vi "pockelscontrol_goMD.vi"() -> ()   [LabVIEW 2012]
doc: "SciScan 1.2 160622"
uses:
  GFG/GFGfpRefGet.vi
  GFG/GFGnumericGet.vi
  GFG/GFGbooleanGet.vi
  GFG/GFGstringGet.vi
  <vilib>/DAQmx/create/channels.llb/DAQmx Create Channel (AO-Voltage-Basic).vi
  <vilib>/DAQmx/write.llb/DAQmx Write (Analog DBL 1Chan 1Samp).vi
  GFG/GFG library.lvlib
panel:
  out "error out 3":errorcluster
  out "error out 2":errorcluster
  out "error out":errorcluster
  out "Source VI":string
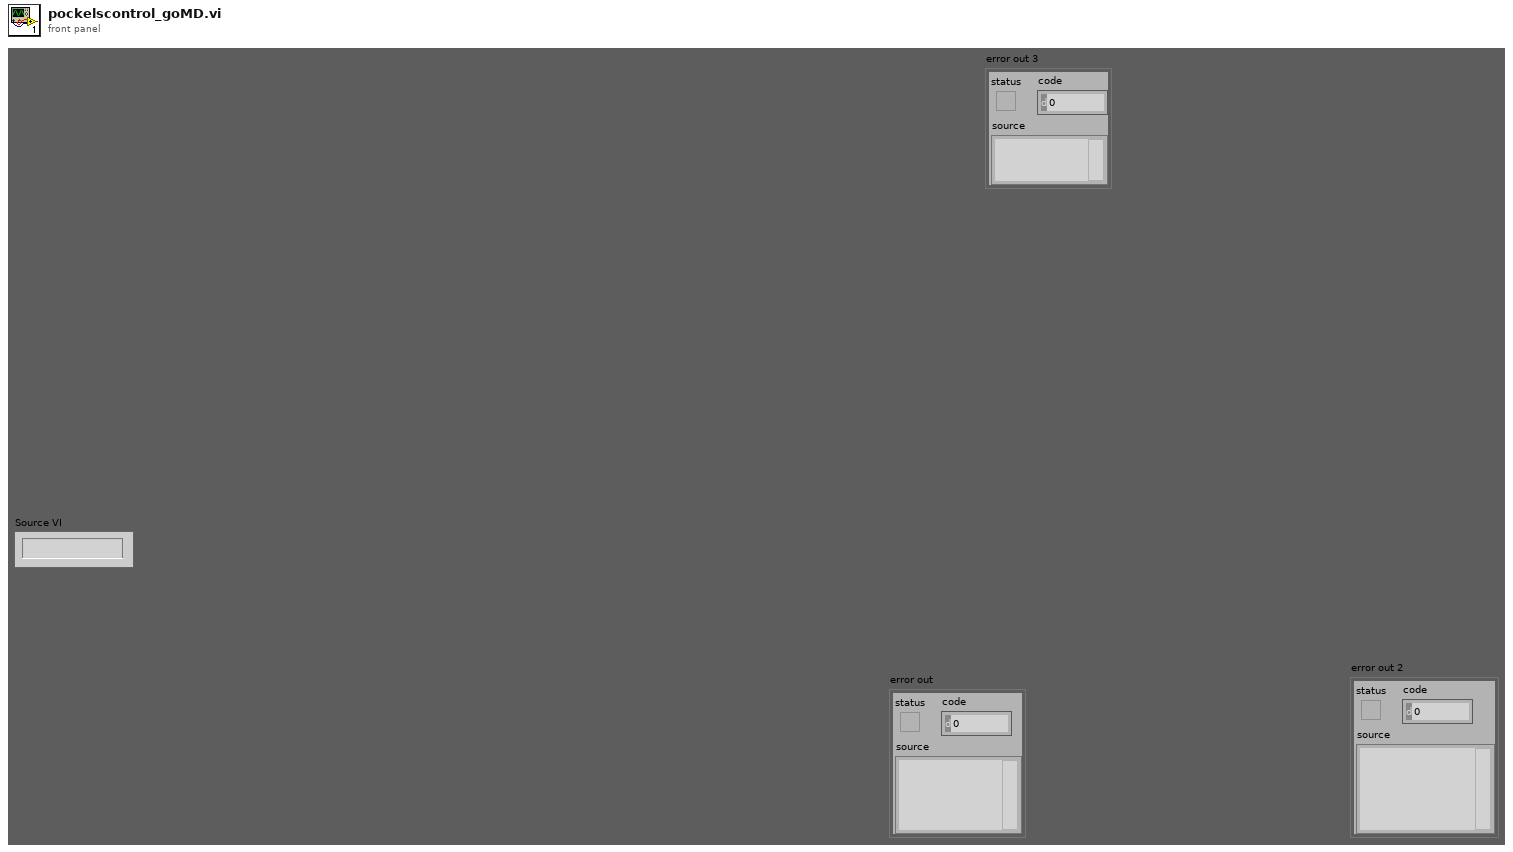
[diagram p1: front panel]
types:
  T1 = enum8{"Enabled", "Disabled", "Disabled and Grayed Out"}
  T2 = cluster{"WaveformChartRef":refnum<vi>, "DigitalRef":refnum<vi>, "ArrayRef":refnum<vi>, "TabControlRef":refnum<vi>, "EnumRef":refnum<vi>, "RingRef":refnum<vi>, "BooleanRef":refnum<vi>, "KnobRef":refnum<vi>, "SlideRef":refnum<vi>, "PathRef":refnum<vi>, "StringRef":refnum<vi>, "ComboBox":refnum<vi>, "WaveformGraphRef":refnum<vi>}
  T3 = enum16{"Left Button", "Center Button", "Right Button", "Window Close"}
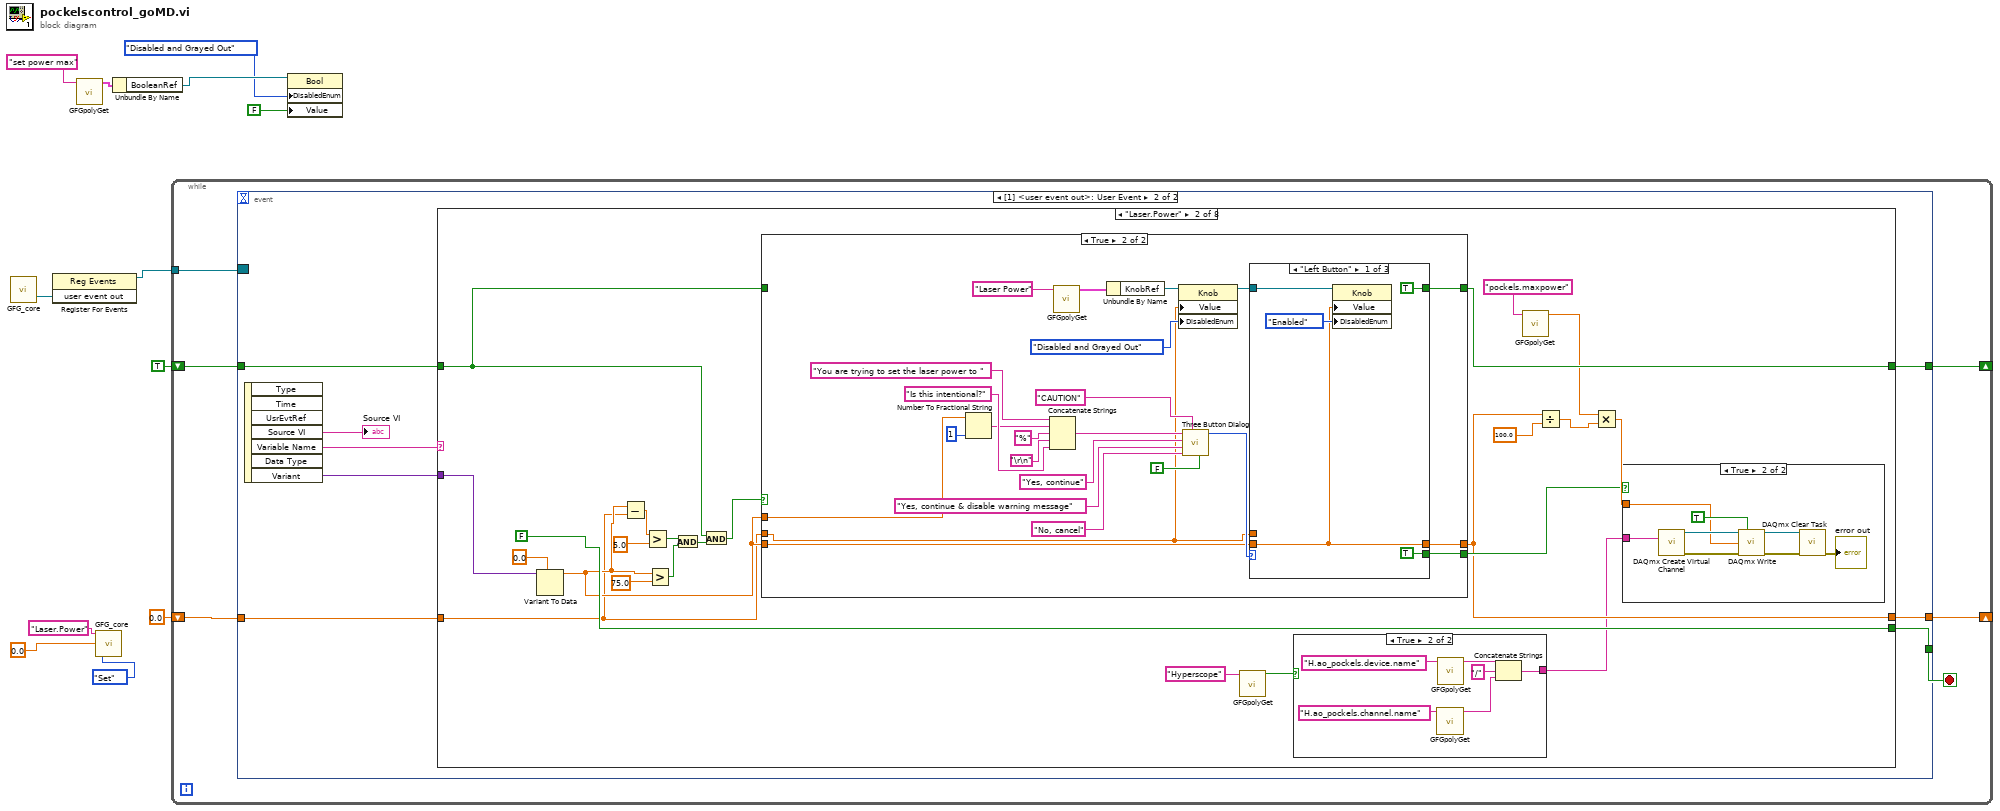
[diagram p0: block diagram]
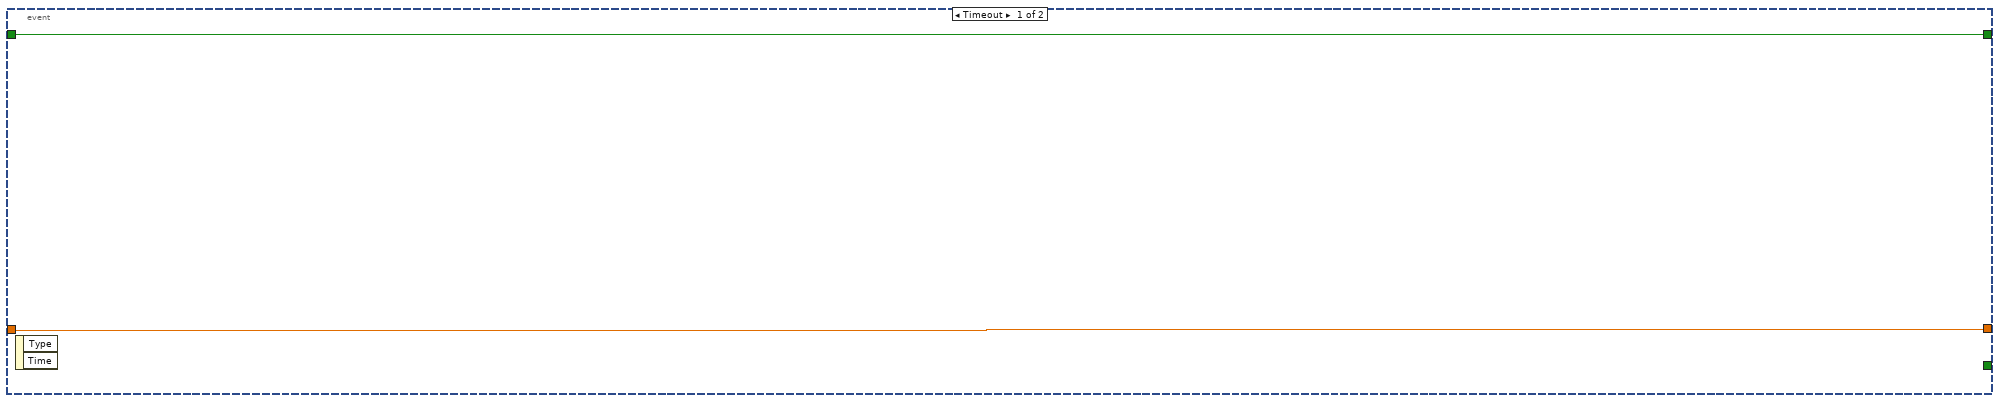
[diagram p2: hidden frame]
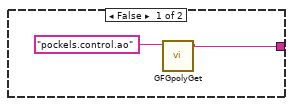
[diagram p4: hidden frame]
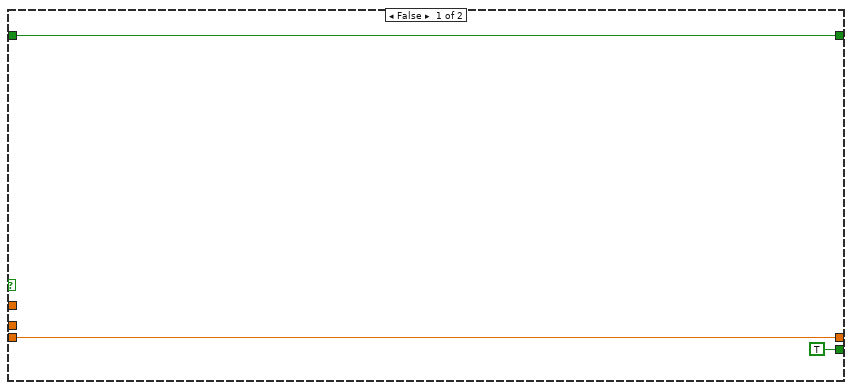
[diagram p5: hidden frame]
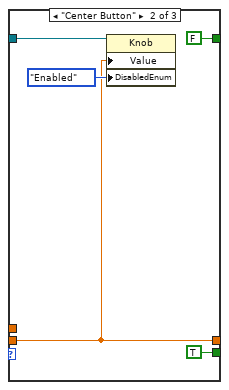
[diagram p6: hidden frame]
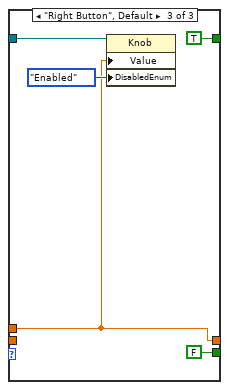
[diagram p7: hidden frame]
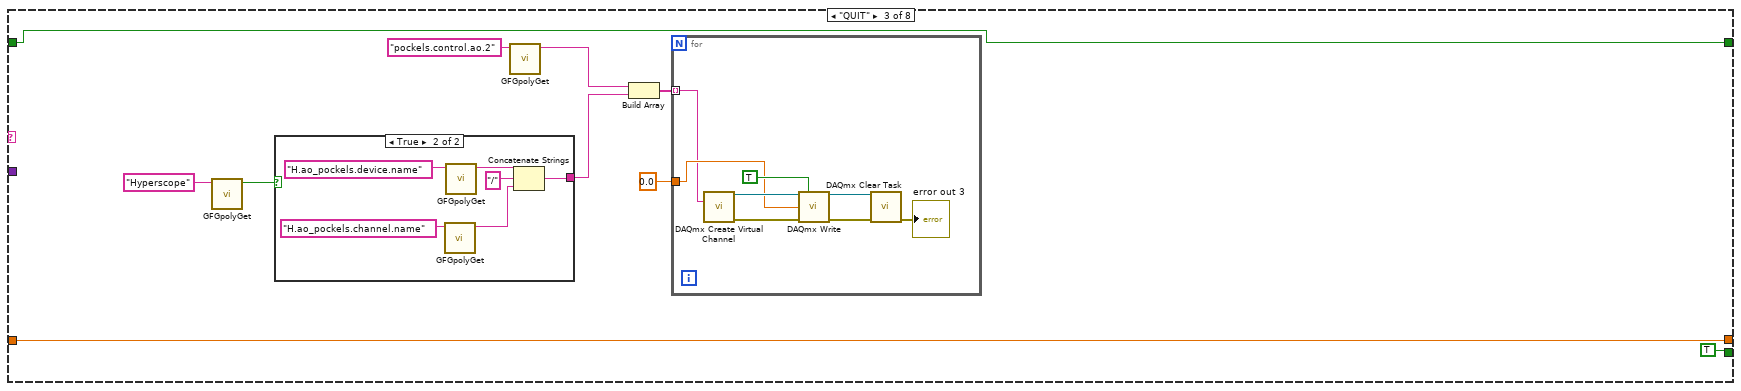
[diagram p9: hidden frame]
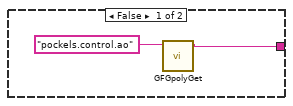
[diagram p10: hidden frame]
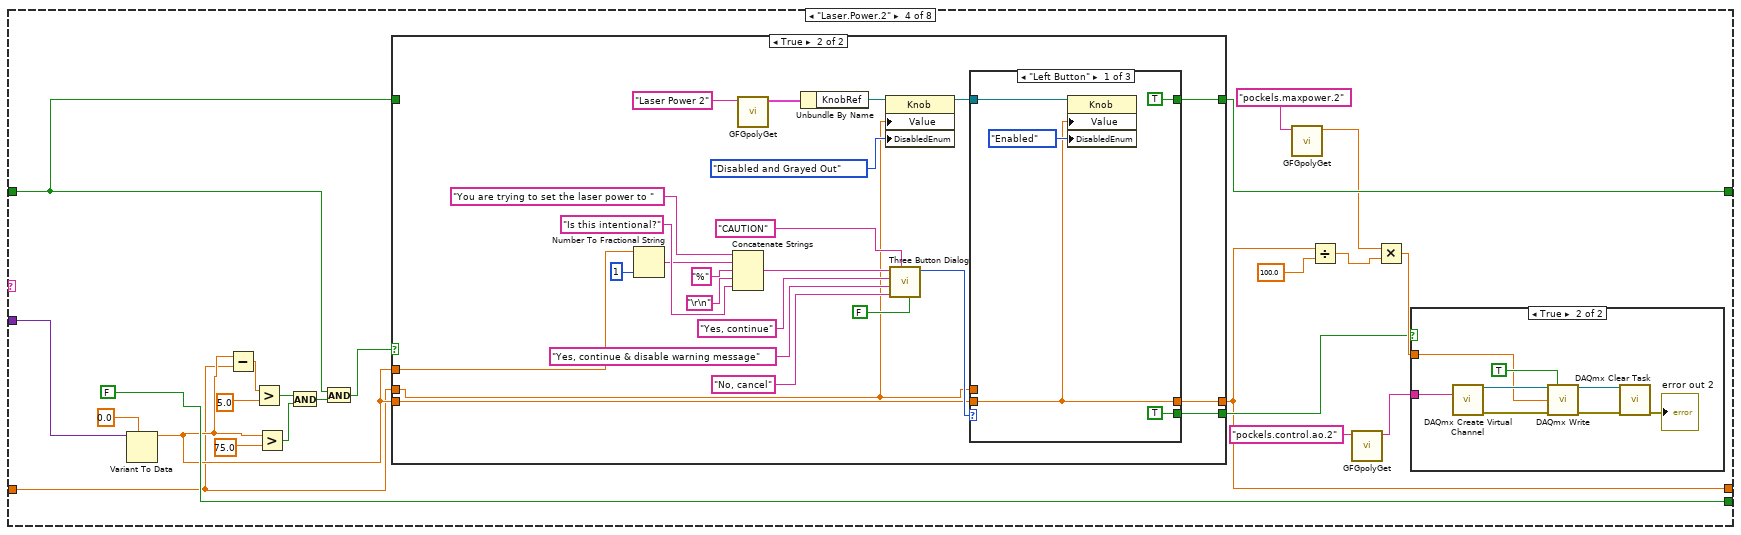
[diagram p11: hidden frame]
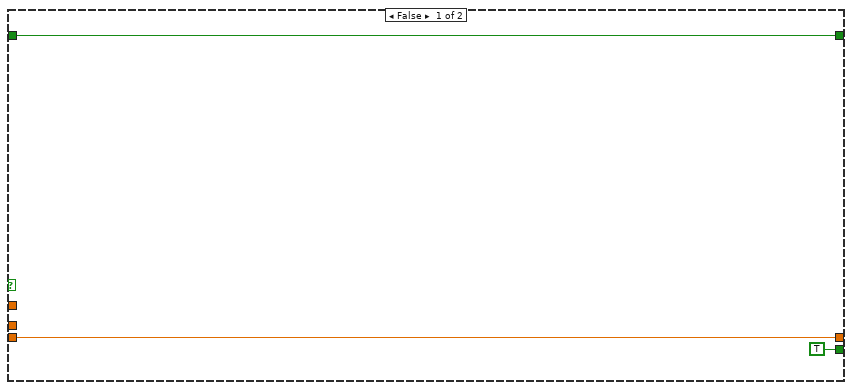
[diagram p12: hidden frame]
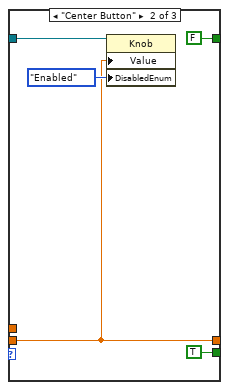
[diagram p13: hidden frame]
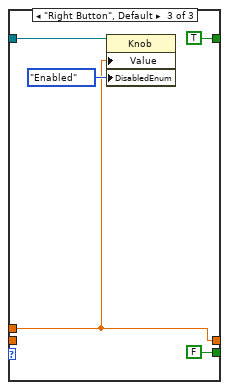
[diagram p14: hidden frame]
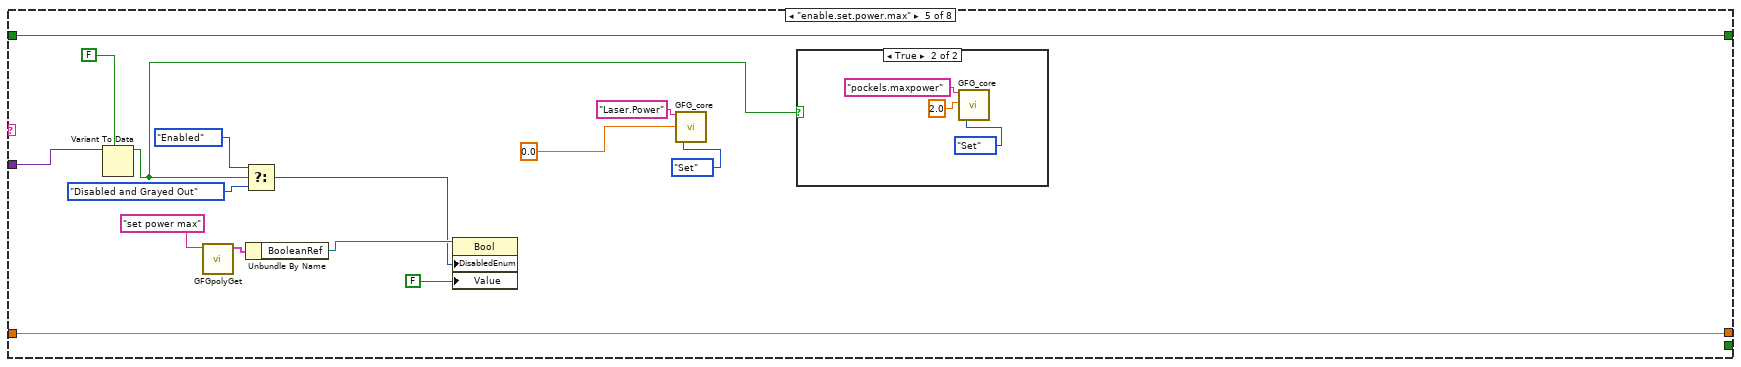
[diagram p16: hidden frame]
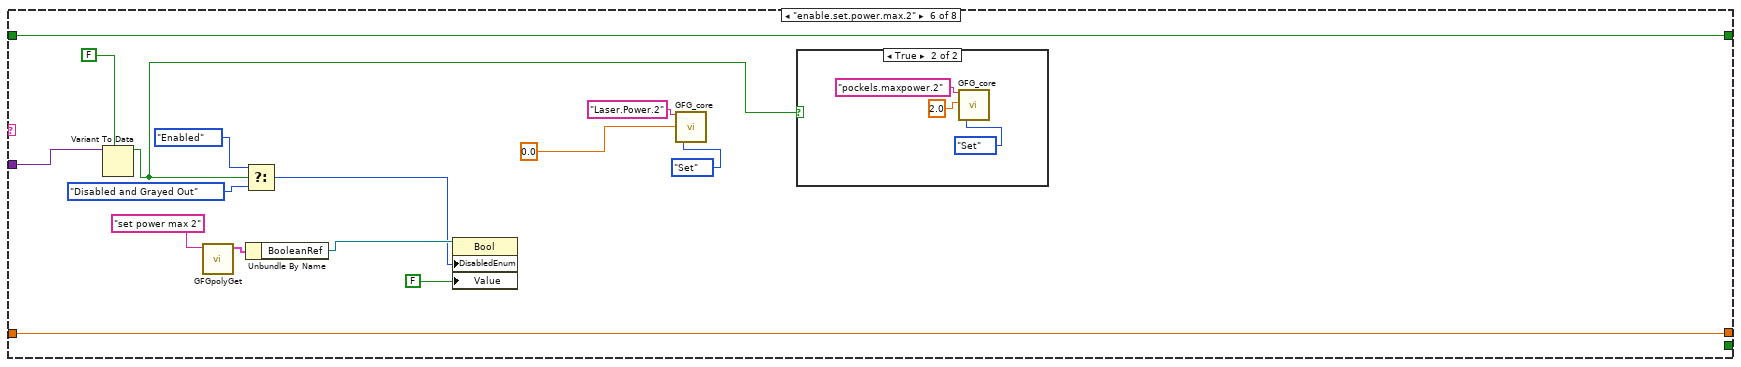
[diagram p18: hidden frame]
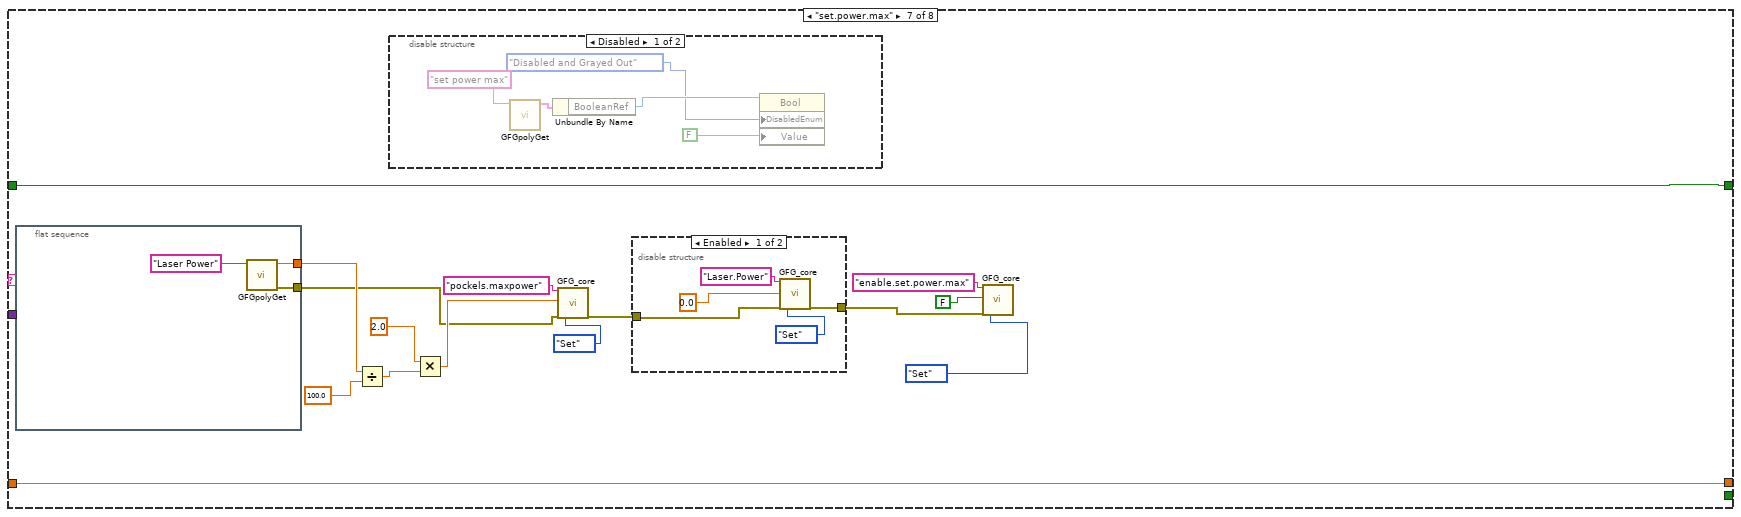
[diagram p20: hidden frame]
diagram:
  n1 = call "GFG_core.vi"() -> ("user event out"=w12:refnum<user-event>)  [unwired: 13 in, 6 out]
  n2 = register-events(w12) -> (reference out=w11:refnum<event-registration>)  [unwired: 2 in, 1 out]
  n3 = call-poly "GFGpolyGet.vi"("Variable Name in"="set power max") -> ("output cluster"=w3:T2)  [unwired: 9 in, 1 out]
  n4 = call "GFG_core.vi"("Variable Name in"="Laser.Power", "Variant in"=0.0 ("Laser Power"), "Action"=enum16{"Init", "Set", "Get"}."Set") -> ()  [unwired: 10 in, 7 out]
  n5 = Unbundle By Name(w3) -> ("BooleanRef"=w4:refnum<vi>)
  n6 = while {
    tunnel: w11 -> [w18]
    shift-right: [w16] -> _
    shift-left: 0.0 ("Laser Power") -> [w15]
    shift-right: [w14] -> _
    shift-left: TRUE -> [w13]
    stop <- w17 stop-if-true
    n7 = event shown="[1] <user event out>: User Event" {
      selector: w18 -> [_ _]
      dyn-events: _ -> [_ _]
      timeout: _ -> [_ _]
      tunnel: [_ w25] -> w17
      tunnel: [w20 w24] -> w16
      tunnel: w15 -> [w20 w23]
      tunnel: [w19 w22] -> w14
      tunnel: w13 -> [w19 w21]
      event Timeout {
        n8 = event-data() -> ()  [unwired: 1 in, 2 out]
      }
      event User Event {
        n9 = event-data() -> ("Source VI"=→"Source VI":string, "Variable Name"=w28:string, "Variant"=w27:variant)  [unwired: 1 in, 4 out]
        n10 = case shown="\"Laser.Power\"" w28 {
          tunnel: w27 -> [_ w54 _ w161 w218 w236 _ _]
          tunnel: [_ FALSE TRUE FALSE _ _ _ _] -> w25
          tunnel: [w30 w43 w117 w150 w223 w241 w262 w290] -> w24
          tunnel: w23 -> [w30 w40 w117 w147 w223 w241 w262 w290]
          tunnel: [w29 w46 w116 w153 w222 w240 w261 w289] -> w22
          tunnel: w21 -> [w29 w44 w116 w151 w222 w240 w261 w289]
          frame "False", Default {
          }
          frame "Laser.Power" {
            n11 = Variant To Data(type=0.0 ("Laser Power"), Variant=w54) -> (data=w41:dbl)  [unwired: 1 in, 1 out]
            n12 = Subtract(x=w41, y=w40) -> (x-y=w39:dbl)
            n13 = Greater?(x=w39, y=5.0) -> (0:w37:bool)
            n14 = Greater?(x=w41, y=75.0) -> (0:w49:bool)
            n15 = And(x=w37, y=w49) -> (x .and. y?=w42:bool)
            n16 = And(x=w44, y=w42) -> (x .and. y?=w45:bool)
            n17 = case shown="True" w45 {
              tunnel: [TRUE w83] -> w47
              tunnel: [w64 w82] -> w46
              tunnel: w44 -> [w64 _]
              tunnel: w40 -> [_ w70]
              tunnel: w41 -> [_ w80]
              tunnel: w41 -> [w63 w71]
              tunnel: [w63 w66] -> w43
              frame False {
              }
              frame True {
                n18 = Number To Fractional String(number=w80, precision (6)=i16 1) -> (F-format string=w69:string)  [unwired: 2 in]
                n19 = Concatenate Strings("You are trying to set the laser power to " ("message"), w69, "%" ("string"), "\r\n", "Is this intentional?" ("string")) -> (w77:string)
                n20 = call-poly "GFGpolyGet.vi"("Variable Name in"="Laser Power") -> ("output cluster"=w75:T2)  [unwired: 9 in, 1 out]
                n21 = Unbundle By Name(w75) -> ("KnobRef"=w74:refnum<vi>)
                n22 = property class="Knob"(reference=w74, "Value"=w70, "DisabledEnum"=T1."Disabled and Grayed Out" ("Disabled")) -> (reference out=w72:refnum<vi>)  [unwired: 1 in, 1 out]
                n23 = call <vilib>:"Three Button Dialog.vi"("Allow user to close window? (TRUE)"=FALSE, "Window Title (\"\")"="CAUTION" ("Window Title (\"\")"), "Right Button Text (\"Cancel\")"="No, cancel" ("Right Button Text (\"Cancel\")"), "Center Button Text (\"No\")"="Yes, continue & disable warning message" ("Center Button Text (\"No\")"), "Left Button Text (\"Yes\")"="Yes, continue" ("Left Button Text (\"Yes\")"), "message"=w77) -> ("Which Button?"=w84:T3)  [unwired: 5 in]
                n24 = case shown="\"Left Button\"" w84 {
                  tunnel: [TRUE TRUE FALSE] -> w83
                  tunnel: [TRUE FALSE TRUE] -> w82
                  tunnel: w72 -> [w91 w96 w101]
                  tunnel: w71 -> [w90 w95 _]
                  tunnel: w70 -> [_ _ w100]
                  tunnel: [w90 w95 w100] -> w66
                  frame "Left Button" {
                    n25 = property class="Knob"(reference=w91, "Value"=w90, "DisabledEnum"=T1."Enabled" ("Disabled")) -> ()  [unwired: 1 in, 2 out]
                  }
                  frame "Center Button" {
                    n26 = property class="Knob"(reference=w96, "Value"=w95, "DisabledEnum"=T1."Enabled" ("Disabled")) -> ()  [unwired: 1 in, 2 out]
                  }
                  frame "Right Button", Default {
                    n27 = property class="Knob"(reference=w101, "Value"=w100, "DisabledEnum"=T1."Enabled" ("Disabled")) -> ()  [unwired: 1 in, 2 out]
                  }
                }
              }
            }
            n28 = call-poly "GFGpolyGet.vi"("Variable Name in"="Hyperscope") -> ("Boolean Value OUT"=w31:bool)  [unwired: 9 in, 1 out]
            n29 = case shown="True" w31 {
              tunnel: [w55 w57] -> w32
              frame False {
                n30 = call-poly "GFGpolyGet.vi"("Variable Name in"="pockels.control.ao" ("Tag in")) -> ("String"=w55:string)  [unwired: 9 in, 1 out]
              }
              frame True {
                n31 = call-poly "GFGpolyGet.vi"("Variable Name in"="H.ao_pockels.channel.name" ("Tag in")) -> ("String"=w58:string)  [unwired: 9 in, 1 out]
                n32 = call-poly "GFGpolyGet.vi"("Variable Name in"="H.ao_pockels.device.name" ("Tag in")) -> ("String"=w61:string)  [unwired: 9 in, 1 out]
                n33 = Concatenate Strings(w61, "/" ("Variable Name in"), w58) -> (w57:string)
              }
            }
            n34 = call-poly "GFGpolyGet.vi"("Variable Name in"="pockels.maxpower") -> ("Numeric"=w35:dbl)  [unwired: 8 in, 2 out]
            n35 = Divide(x=w43, y=100.0 ("x")) -> (x/y=w52:dbl)
            n36 = Multiply(x=w35, y=w52) -> (x*y=w50:dbl)
            n37 = case shown="True" w47 {
              tunnel: w32 -> [_ w112]
              tunnel: w50 -> [_ w106]
              frame False {
              }
              frame True {
                n38 = call-poly <vilib>:"DAQmx Create Virtual Channel.vi"("physical channels"=w112) -> ("task out"=w111:refnum<k21>, "error out"=w107:errorcluster)  [unwired: 13 in]
                n39 = call-poly <vilib>:"DAQmx Write.vi"("task/channels in"=w111, "auto start"=TRUE, "data"=w106, "error in"=w107) -> ("task out"=w109:refnum<k21>, "error out"=w108:errorcluster)  [unwired: 9 in, 1 out]
                n40 = call <vilib>:"DAQmx Clear Task.vi"("task in"=w109, "error in"=w108) -> ("error out"=→"error out":errorcluster)  [unwired: 13 in]
              }
            }
          }
          frame "QUIT" {
            n41 = call-poly "GFGpolyGet.vi"("Variable Name in"="Hyperscope") -> ("Boolean Value OUT"=w113:bool)  [unwired: 9 in, 1 out]
            n42 = case shown="True" w113 {
              tunnel: [w123 w125] -> w114
              frame False {
                n43 = call-poly "GFGpolyGet.vi"("Variable Name in"="pockels.control.ao" ("Tag in")) -> ("String"=w123:string)  [unwired: 9 in, 1 out]
              }
              frame True {
                n44 = call-poly "GFGpolyGet.vi"("Variable Name in"="H.ao_pockels.channel.name" ("Tag in")) -> ("String"=w126:string)  [unwired: 9 in, 1 out]
                n45 = call-poly "GFGpolyGet.vi"("Variable Name in"="H.ao_pockels.device.name" ("Tag in")) -> ("String"=w129:string)  [unwired: 9 in, 1 out]
                n46 = Concatenate Strings(w129, "/" ("Variable Name in"), w126) -> (w125:string)
              }
            }
            n47 = call-poly "GFGpolyGet.vi"("Variable Name in"="pockels.control.ao.2" ("Tag in")) -> ("String"=w120:string)  [unwired: 9 in, 1 out]
            n48 = Build Array(w120, w114) -> (w119:string[])
            n49 = for {
              tunnel: 0.0 ("data") -> [w132]
              tunnel: w119 -> [w131] mode=indexing
              n50 = call-poly <vilib>:"DAQmx Create Virtual Channel.vi"("physical channels"=w131) -> ("task out"=w138:refnum<k21>, "error out"=w134:errorcluster)  [unwired: 13 in]
              n51 = call-poly <vilib>:"DAQmx Write.vi"("task/channels in"=w138, "auto start"=TRUE, "data"=w132, "error in"=w134) -> ("task out"=w136:refnum<k21>, "error out"=w135:errorcluster)  [unwired: 9 in, 1 out]
              n52 = call <vilib>:"DAQmx Clear Task.vi"("task in"=w136, "error in"=w135) -> ("error out"=→"error out 3":errorcluster)  [unwired: 13 in]
            }
          }
          frame "Laser.Power.2" {
            n53 = Variant To Data(type=0.0 ("Laser Power"), Variant=w161) -> (data=w148:dbl)  [unwired: 1 in, 1 out]
            n54 = Subtract(x=w148, y=w147) -> (x-y=w146:dbl)
            n55 = Greater?(x=w146, y=5.0) -> (0:w144:bool)
            n56 = Greater?(x=w148, y=75.0) -> (0:w156:bool)
            n57 = And(x=w144, y=w156) -> (x .and. y?=w149:bool)
            n58 = And(x=w151, y=w149) -> (x .and. y?=w152:bool)
            n59 = case shown="True" w152 {
              tunnel: [TRUE w182] -> w154
              tunnel: [w163 w181] -> w153
              tunnel: w151 -> [w163 _]
              tunnel: w147 -> [_ w169]
              tunnel: w148 -> [_ w179]
              tunnel: w148 -> [w162 w170]
              tunnel: [w162 w165] -> w150
              frame False {
              }
              frame True {
                n60 = Number To Fractional String(number=w179, precision (6)=i16 1) -> (F-format string=w168:string)  [unwired: 2 in]
                n61 = Concatenate Strings("You are trying to set the laser power to " ("message"), w168, "%" ("string"), "\r\n", "Is this intentional?" ("string")) -> (w176:string)
                n62 = call-poly "GFGpolyGet.vi"("Variable Name in"="Laser Power 2") -> ("output cluster"=w174:T2)  [unwired: 9 in, 1 out]
                n63 = Unbundle By Name(w174) -> ("KnobRef"=w173:refnum<vi>)
                n64 = property class="Knob"(reference=w173, "Value"=w169, "DisabledEnum"=T1."Disabled and Grayed Out" ("Disabled")) -> (reference out=w171:refnum<vi>)  [unwired: 1 in, 1 out]
                n65 = call <vilib>:"Three Button Dialog.vi"("Allow user to close window? (TRUE)"=FALSE, "Window Title (\"\")"="CAUTION" ("Window Title (\"\")"), "Right Button Text (\"Cancel\")"="No, cancel" ("Right Button Text (\"Cancel\")"), "Center Button Text (\"No\")"="Yes, continue & disable warning message" ("Center Button Text (\"No\")"), "Left Button Text (\"Yes\")"="Yes, continue" ("Left Button Text (\"Yes\")"), "message"=w176) -> ("Which Button?"=w183:T3)  [unwired: 5 in]
                n66 = case shown="\"Left Button\"" w183 {
                  tunnel: [TRUE TRUE FALSE] -> w182
                  tunnel: [TRUE FALSE TRUE] -> w181
                  tunnel: w171 -> [w190 w195 w200]
                  tunnel: w170 -> [w189 w194 _]
                  tunnel: w169 -> [_ _ w199]
                  tunnel: [w189 w194 w199] -> w165
                  frame "Left Button" {
                    n67 = property class="Knob"(reference=w190, "Value"=w189, "DisabledEnum"=T1."Enabled" ("Disabled")) -> ()  [unwired: 1 in, 2 out]
                  }
                  frame "Center Button" {
                    n68 = property class="Knob"(reference=w195, "Value"=w194, "DisabledEnum"=T1."Enabled" ("Disabled")) -> ()  [unwired: 1 in, 2 out]
                  }
                  frame "Right Button", Default {
                    n69 = property class="Knob"(reference=w200, "Value"=w199, "DisabledEnum"=T1."Enabled" ("Disabled")) -> ()  [unwired: 1 in, 2 out]
                  }
                }
              }
            }
            n70 = call-poly "GFGpolyGet.vi"("Variable Name in"="pockels.maxpower.2") -> ("Numeric"=w142:dbl)  [unwired: 8 in, 2 out]
            n71 = Divide(x=w150, y=100.0 ("x")) -> (x/y=w159:dbl)
            n72 = call-poly "GFGpolyGet.vi"("Variable Name in"="pockels.control.ao.2" ("Tag in")) -> ("String"=w140:string)  [unwired: 9 in, 1 out]
            n73 = Multiply(x=w142, y=w159) -> (x*y=w157:dbl)
            n74 = case shown="True" w154 {
              tunnel: w140 -> [_ w211]
              tunnel: w157 -> [_ w205]
              frame False {
              }
              frame True {
                n75 = call-poly <vilib>:"DAQmx Create Virtual Channel.vi"("physical channels"=w211) -> ("task out"=w210:refnum<k21>, "error out"=w206:errorcluster)  [unwired: 13 in]
                n76 = call-poly <vilib>:"DAQmx Write.vi"("task/channels in"=w210, "auto start"=TRUE, "data"=w205, "error in"=w206) -> ("task out"=w208:refnum<k21>, "error out"=w207:errorcluster)  [unwired: 9 in, 1 out]
                n77 = call <vilib>:"DAQmx Clear Task.vi"("task in"=w208, "error in"=w207) -> ("error out"=→"error out 2":errorcluster)  [unwired: 13 in]
              }
            }
          }
          frame "enable.set.power.max" {
            n78 = Variant To Data(type=FALSE, Variant=w218) -> (data=w213:bool)  [unwired: 1 in, 1 out]
            n79 = call-poly "GFGpolyGet.vi"("Variable Name in"="set power max") -> ("output cluster"=w225:T2)  [unwired: 9 in, 1 out]
            n80 = Select(t=T1."Enabled" ("Disabled"), s=w213, f=T1."Disabled and Grayed Out" ("Disabled")) -> (s? t:f=w214:T1)
            n81 = Unbundle By Name(w225) -> ("BooleanRef"=w224:refnum<vi>)
            n82 = property class="Bool"(reference=w224, "DisabledEnum"=w214, "Value"=FALSE) -> ()  [unwired: 1 in, 2 out]
            n83 = call "GFG_core.vi"("Variable Name in"="Laser.Power", "Variant in"=0.0 ("Laser Power"), "Action"=enum16{"Init", "Set", "Get"}."Set") -> ()  [unwired: 10 in, 7 out]
            n84 = case shown="True" w213 {
              frame False {
              }
              frame True {
                n85 = call "GFG_core.vi"("Variable Name in"="pockels.maxpower", "Variant in"=2.0 ("Laser Power"), "Action"=enum16{"Init", "Set", "Get"}."Set") -> ()  [unwired: 10 in, 7 out]
              }
            }
          }
          frame "enable.set.power.max.2" {
            n86 = Variant To Data(type=FALSE, Variant=w236) -> (data=w231:bool)  [unwired: 1 in, 1 out]
            n87 = call-poly "GFGpolyGet.vi"("Variable Name in"="set power max 2") -> ("output cluster"=w243:T2)  [unwired: 9 in, 1 out]
            n88 = Select(t=T1."Enabled" ("Disabled"), s=w231, f=T1."Disabled and Grayed Out" ("Disabled")) -> (s? t:f=w232:T1)
            n89 = Unbundle By Name(w243) -> ("BooleanRef"=w242:refnum<vi>)
            n90 = property class="Bool"(reference=w242, "DisabledEnum"=w232, "Value"=FALSE) -> ()  [unwired: 1 in, 2 out]
            n91 = call "GFG_core.vi"("Variable Name in"="Laser.Power.2", "Variant in"=0.0 ("Laser Power"), "Action"=enum16{"Init", "Set", "Get"}."Set") -> ()  [unwired: 10 in, 7 out]
            n92 = case shown="True" w231 {
              frame False {
              }
              frame True {
                n93 = call "GFG_core.vi"("Variable Name in"="pockels.maxpower.2", "Variant in"=2.0 ("Laser Power"), "Action"=enum16{"Init", "Set", "Get"}."Set") -> ()  [unwired: 10 in, 7 out]
              }
            }
          }
          frame "set.power.max" {
            n94 = flat-sequence {
              tunnel: [w269] -> w257
              tunnel: [w268] -> w253
              frame #0 {
                n95 = call-poly "GFGpolyGet.vi"("Variable Name in"="Laser Power") -> ("error out"=w268:errorcluster, "Numeric"=w269:dbl)  [unwired: 8 in, 1 out]
              }
            }
            n96 = Divide(x=w257, y=100.0 ("x")) -> (x/y=w256:dbl)
            n97 = disable-structure shown="Disabled" {
              frame Disabled {
                n98 = call-poly "GFGpolyGet.vi"("Variable Name in"="set power max") -> ("output cluster"=w274:T2)  [unwired: 9 in, 1 out]
                n99 = Unbundle By Name(w274) -> ("BooleanRef"=w273:refnum<vi>)
                n100 = property class="Bool"(reference=w273, "DisabledEnum"=T1."Disabled and Grayed Out" ("Disabled"), "Value"=FALSE) -> ()  [unwired: 1 in, 2 out]
              }
              frame Enabled {
              }
            }
            n101 = Multiply(x=2.0 ("Laser Power"), y=w256) -> (x*y=w254:dbl)
            n102 = call "GFG_core.vi"("Variable Name in"="pockels.maxpower", "Variant in"=w254, "error in (no error)"=w253, "Action"=enum16{"Init", "Set", "Get"}."Set") -> ("error out"=w252:errorcluster)  [unwired: 9 in, 6 out]
            n103 = disable-structure shown="Enabled" {
              disable-tunnel: w252 -> [w264 _]
              disable-tunnel: [w263 _] -> w249
              frame Enabled {
                n104 = call "GFG_core.vi"("Variable Name in"="Laser.Power", "Variant in"=0.0 ("Laser Power"), "error in (no error)"=w264, "Action"=enum16{"Init", "Set", "Get"}."Set") -> ("error out"=w263:errorcluster)  [unwired: 9 in, 6 out]
              }
              frame Disabled {
              }
            }
            n105 = call "GFG_core.vi"("Variable Name in"="enable.set.power.max", "Variant in"=FALSE, "error in (no error)"=w249, "Action"=enum16{"Init", "Set", "Get"}."Set") -> ()  [unwired: 9 in, 7 out]
          }
          frame "set.power.max.2" {
            n106 = flat-sequence {
              tunnel: [w297] -> w285
              tunnel: [w296] -> w281
              frame #0 {
                n107 = call-poly "GFGpolyGet.vi"("Variable Name in"="Laser Power 2") -> ("error out"=w296:errorcluster, "Numeric"=w297:dbl)  [unwired: 8 in, 1 out]
              }
            }
            n108 = Divide(x=w285, y=100.0 ("x")) -> (x/y=w284:dbl)
            n109 = disable-structure shown="Disabled" {
              frame Disabled {
                n110 = call-poly "GFGpolyGet.vi"("Variable Name in"="set power max") -> ("output cluster"=w302:T2)  [unwired: 9 in, 1 out]
                n111 = Unbundle By Name(w302) -> ("BooleanRef"=w301:refnum<vi>)
                n112 = property class="Bool"(reference=w301, "DisabledEnum"=T1."Disabled and Grayed Out" ("Disabled"), "Value"=FALSE) -> ()  [unwired: 1 in, 2 out]
              }
              frame Enabled {
              }
            }
            n113 = Multiply(x=2.0 ("Laser Power"), y=w284) -> (x*y=w282:dbl)
            n114 = call "GFG_core.vi"("Variable Name in"="pockels.maxpower.2", "Variant in"=w282, "error in (no error)"=w281, "Action"=enum16{"Init", "Set", "Get"}."Set") -> ("error out"=w280:errorcluster)  [unwired: 9 in, 6 out]
            n115 = disable-structure shown="Enabled" {
              disable-tunnel: w280 -> [w292 _]
              disable-tunnel: [w291 _] -> w277
              frame Enabled {
                n116 = call "GFG_core.vi"("Variable Name in"="Laser.Power.2", "Variant in"=0.0 ("Laser Power"), "error in (no error)"=w292, "Action"=enum16{"Init", "Set", "Get"}."Set") -> ("error out"=w291:errorcluster)  [unwired: 9 in, 6 out]
              }
              frame Disabled {
              }
            }
            n117 = call "GFG_core.vi"("Variable Name in"="enable.set.power.max.2", "Variant in"=FALSE, "error in (no error)"=w277, "Action"=enum16{"Init", "Set", "Get"}."Set") -> ()  [unwired: 9 in, 7 out]
          }
        }
      }
    }
  }
  n118 = property class="Bool"(reference=w4, "DisabledEnum"=T1."Disabled and Grayed Out" ("Disabled"), "Value"=FALSE) -> ()  [unwired: 1 in, 2 out]
